vi "FindItem.vi"(8 "error in":errorcluster, 10 "Items":string[](array[string]), 11 "GObj Refnum":refnum<vi>) -> (0 "error out":errorcluster, 1 "Reject?":bool, 2 "Identifier":string, 3 "dup GObj Refnum":refnum<vi>)   [LabVIEW 2015, in "lvbuildsecurity.lvlib" / "Invoke.lvclass"]
uses:
  Invoke.lvclass
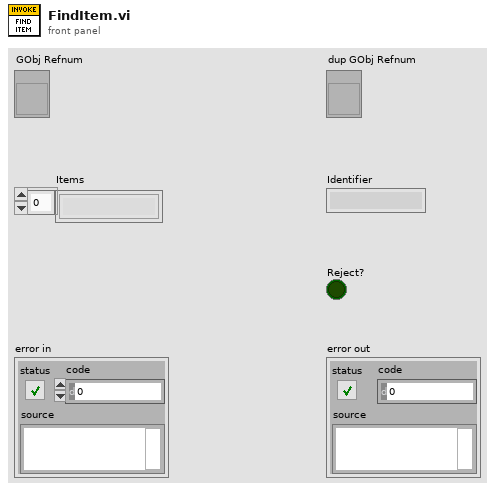
[diagram p1: front panel]
types:
  T1 = typedef "ASPM_UniqueIDStringDatanameShortnameLongname.ctl" = cluster{"Unique ID string":string, "Data name":string, "Short name (localized)":string, "Long name (localized)":string}
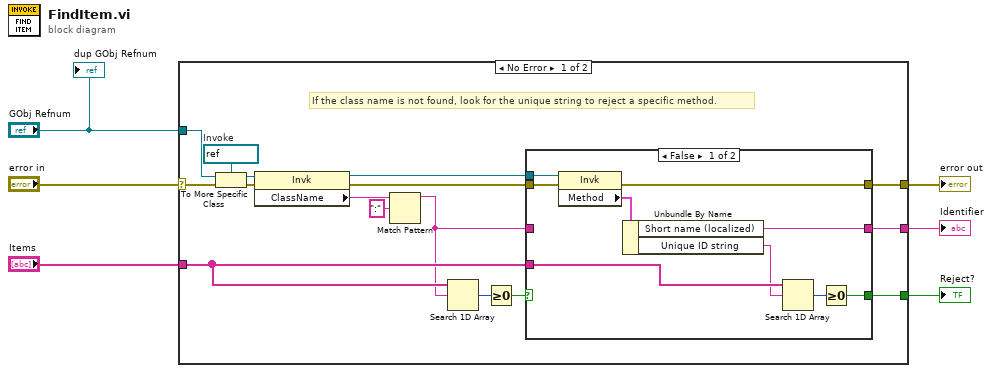
[diagram p0: block diagram]
diagram:
  n1 = case shown="No Error" "error in" {
    selector: "error in" -> [w7 w35]
    tunnel: "GObj Refnum" -> [w16 _]
    tunnel: "Items" -> [w12 _]
    tunnel: [w10 _] -> w4
    tunnel: [w9 _] -> w3
    tunnel: [w8 w35] -> w2
    frame No Error {
      w22 = refnum<vi> refnum  # Invoke
      # "If the class name is not found, look for the unique string to reject a specific method."
      n2 = To More Specific Class(target class=w22, reference=w16, error in=w7) -> (specific class reference=w20:refnum<vi>, error out=w21:errorcluster)
      n3 = property class="Invk"(reference=w20, error in=w21) -> (reference out=w14:refnum<vi>, error out=w13:errorcluster, "ClassName"=w17:string)
      n4 = Match Pattern(string=w17, regular expression=":") -> (before substring=w11:string)  [unwired: 1 in, 3 out]
      n5 = Search 1D Array(1D array=w12, element=w11) -> (index of element=w19:i32)  [unwired: 1 in]
      n6 = Greater Or Equal To 0?(x=w19) -> (x >= 0?=w15:bool)
      n7 = case shown="False" w15 {
        selector: w15 -> [_ w34]
        tunnel: w14 -> [w31 _]
        tunnel: w13 -> [w30 w32]
        tunnel: w12 -> [w27 _]
        tunnel: [w25 w34] -> w10
        tunnel: w11 -> [_ w33]
        tunnel: [w24 w33] -> w9
        tunnel: [w23 w32] -> w8
        frame False {
          n8 = property class="Invk"(reference=w31, error in=w30) -> (error out=w23:errorcluster, "Method"=w29:T1)  [unwired: 1 out]
          n9 = Unbundle By Name(w29) -> ("Short name (localized)"=w24:string, "Unique ID string"=w26:string)
          n10 = Search 1D Array(1D array=w27, element=w26) -> (index of element=w28:i32)  [unwired: 1 in]
          n11 = Greater Or Equal To 0?(x=w28) -> (x >= 0?=w25:bool)
        }
        frame True {
        }
      }
    }
    frame Error {
    }
  }
  "Reject?" <- w4
  "Identifier" <- w3
  "error out" <- w2
  "dup GObj Refnum" <- "GObj Refnum"
